vi "Aula 21_09TR-TC.vi"(11 "TR":dbl) -> (3 "TC":dbl)   [LabVIEW 2020]
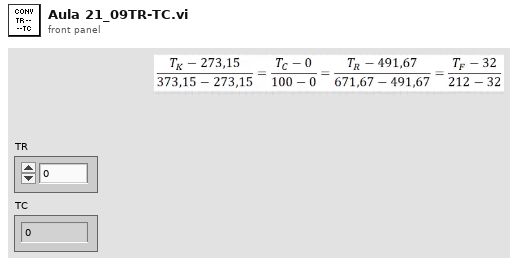
[diagram p1: front panel]
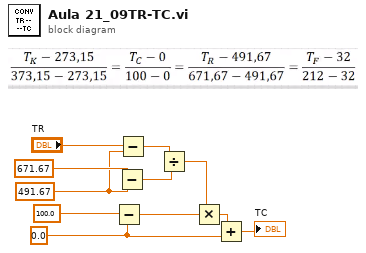
[diagram p0: block diagram]
diagram:
  w1 = 491.67 ("x*y")
  w7 = 0.0 ("y")
  n1 = Subtract(x=100.0 ("y"), y=w7) -> (x-y=w9:dbl)
  n2 = Subtract(x=671.67 ("y"), y=w1) -> (x-y=w5:dbl)
  n3 = Subtract(x="TR", y=w1) -> (x-y=w4:dbl)
  n4 = Divide(x=w4, y=w5) -> (x/y=w3:dbl)
  n5 = Multiply(x=w3, y=w9) -> (x*y=w8:dbl)
  n6 = Add(x=w8, y=w7) -> (x+y=→"TC":dbl)
